vi "clearArray_test.vi"() -> ()   [LabVIEW 2014]
panel:
  out "IsEmpty 3":bool
  out "IsEmpty 2":bool
  out "IsEmpty":bool
  out "Out czyszczony":i32[](array[numeric])
  out "Out tak jak in":i32[](array[numeric])
  out "Out Empty":i32[](array[numeric])
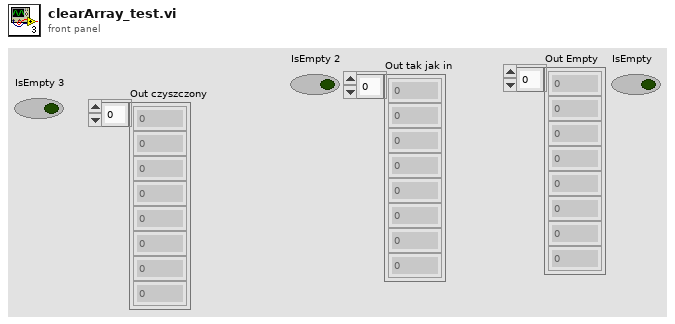
[diagram p1: front panel]
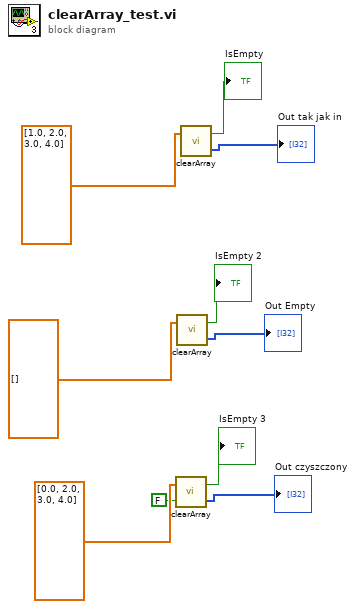
[diagram p0: block diagram]
diagram:
  n1 = call "clearArray.vi"("isActive"=FALSE, "In"=dbl[] [0.0, 2.0, 3.0, 4.0]) -> ("Out"=→"Out czyszczony":i32[], "IsEmpty"=→"IsEmpty 3":bool)
  n2 = call "clearArray.vi"("In"=dbl[] []) -> ("Out"=→"Out Empty":i32[], "IsEmpty"=→"IsEmpty 2":bool)  [unwired: 1 in]
  n3 = call "clearArray.vi"("In"=dbl[] [1.0, 2.0, 3.0, 4.0]) -> ("Out"=→"Out tak jak in":i32[], "IsEmpty"=→"IsEmpty":bool)  [unwired: 1 in]
